vi "Plot Data.vi"(7 "Max Value":dbl, 11 "Data":dbl[][](array[numeric])) -> (3 "XY Graph":cluster{"X":dbl, "Y":dbl}[](array[cluster]))   [LabVIEW 2016]
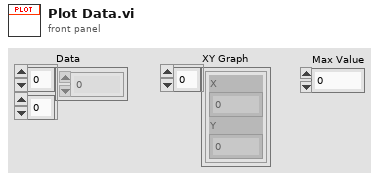
[diagram p1: front panel]
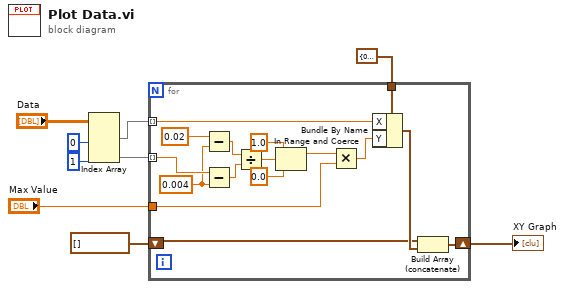
[diagram p0: block diagram]
diagram:
  n1 = Index Array(array="Data", index (col) #1=0 ("disabled index (col)"), index (col) #2=1 ("index (col)")) -> (element #1=w4:dbl[], element #2=w2:dbl[])  [unwired: 2 in]
  n2 = for {
    tunnel: w2 -> [w20] mode=indexing
    shift-right: [w22] -> w9
    shift-left: cluster{"X":dbl, "Y":dbl}[] [] ("Thermocouple 1") -> [w23]
    tunnel: cluster{"X":dbl, "Y":dbl} {"X"=0.0, "Y"=0.0} -> [w25]
    tunnel: w4 -> [w21] mode=indexing
    tunnel: "Max Value" -> [w11]
    w18 = 0.004 ("y")
    n3 = Subtract(x=0.02 ("y"), y=w18) -> (x-y=w16:dbl)
    n4 = Subtract(x=w20, y=w18) -> (x-y=w19:dbl)
    n5 = Divide(x=w16, y=w19) -> (x/y=w15:dbl)
    n6 = In Range and Coerce(upper limit=1.0, x=w15, lower limit=0.0) -> (coerced(x)=w12:dbl)  [unwired: 1 out]
    n7 = Multiply(x=w12, y=w11) -> (x*y=w10:dbl)
    n8 = Bundle By Name(cluster=w25, "X"=w21, "Y"=w10) -> (w24:cluster{"X":dbl, "Y":dbl})
    n9 = Build Array (concatenate)(w23, w24) -> (w22:cluster{"X":dbl, "Y":dbl}[])
  }
  "XY Graph" <- w9
